vi "Write Cell Status File.vi"(7 "Cell Select":i32, 9 "GenInfoIn":T1, 10 "Test Info":T2 {"Cell Data"."Rw Temp" format="%.2f"; "Cell Data"."Rw" format="%.2f"; "Cell Data"."DAQ Units" items=["Mins", "Hrs"]; "Cell Data"."CurData" format="%.3f"; "Cell Data"."Last Pore Vol" format="%.3f"; "Cell Data"."Amplitude" format="%.3f"; "Cell Data"."ElectSpace" format="%.2f"; "Cell Data"."Permeability" format="%.2f"; "Cell Data"."Porosity" format="%.2f"; "Cell Data"."Diameter" format="%.2f"; "Cell Data"."Length" format="%.2f"}, 11 "Filepath":path) -> (3 "FilePathOut":path)   [LabVIEW 2013]
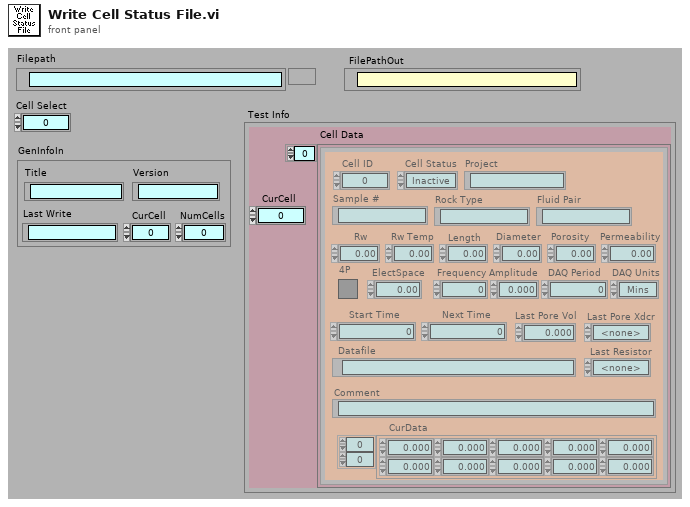
[diagram p1: front panel]
types:
  T1 = cluster{"Title":string, "Version":string, "Last Write":string, "CurCell":i32, "NumCells":i32}
  T2 = cluster{"CurCell":i32, "Cell Data":cluster{"Cell ID":i32, "Cell Status":enum16{"Inactive", "Setup", "Active", "Done"}, "Project":string, "Sample #":string, "Rock Type":string, "Fluid Pair":string, "Rw":dbl, "Rw Temp":dbl, "Length":dbl, "Diameter":dbl, "Porosity":dbl, "Permeability":dbl, "4P":bool, "ElectSpace":dbl, "Frequency":dbl, "Amplitude":dbl, "DAQ Period":u32, "DAQ Units":u16, "Start Time":dbl, "Next Time":dbl, "Datafile":path, "Last Pore Vol":dbl, "Last Pore Xdcr":enum16{"<none>", "Lo Range", "Hi Range"}, "Last Resistor":enum16{"<none>", "Resistor 1", "Resistor 2", "Resistor 3", "Resistor 4", "Resistor 5", "Resistor 6"}, "CurData":dbl[][], "Comment":string}[]}
  T3 = enum16{"New File", "Read Cell Status", "Write Cell Status"}
  T4 = cluster{"Cell ID":i32, "Cell Status":enum16{"Inactive", "Setup", "Active", "Done"}, "Project":string, "Sample #":string, "Rock Type":string, "Fluid Pair":string, "Rw":dbl, "Rw Temp":dbl, "Length":dbl, "Diameter":dbl, "Porosity":dbl, "Permeability":dbl, "4P":bool, "ElectSpace":dbl, "Frequency":dbl, "Amplitude":dbl, "DAQ Period":u32, "DAQ Units":u16, "Start Time":dbl, "Next Time":dbl, "Datafile":path, "Last Pore Vol":dbl, "Last Pore Xdcr":enum16{"<none>", "Lo Range", "Hi Range"}, "Last Resistor":enum16{"<none>", "Resistor 1", "Resistor 2", "Resistor 3", "Resistor 4", "Resistor 5", "Resistor 6"}, "CurData":dbl[][], "Comment":string}[]
  T5 = cluster{"Cell ID":i32, "Cell Status":enum16{"Inactive", "Setup", "Active", "Done"}, "Project":string, "Sample #":string, "Rock Type":string, "Fluid Pair":string, "Rw":dbl, "Rw Temp":dbl, "Length":dbl, "Diameter":dbl, "Porosity":dbl, "Permeability":dbl, "4P":bool, "ElectSpace":dbl, "Frequency":dbl, "Amplitude":dbl, "DAQ Period":u32, "DAQ Units":u16, "Start Time":dbl, "Next Time":dbl, "Datafile":path, "Last Pore Vol":dbl, "Last Pore Xdcr":enum16{"<none>", "Lo Range", "Hi Range"}, "Last Resistor":enum16{"<none>", "Resistor 1", "Resistor 2", "Resistor 3", "Resistor 4", "Resistor 5", "Resistor 6"}, "CurData":dbl[][], "Comment":string}
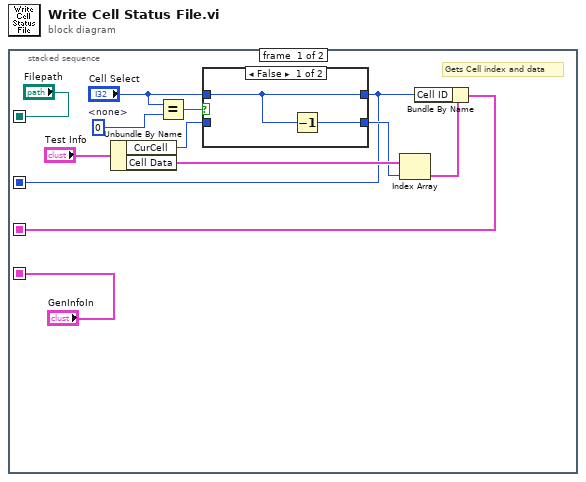
[diagram p0: block diagram]
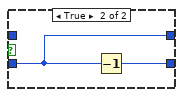
[diagram p2: hidden frame]
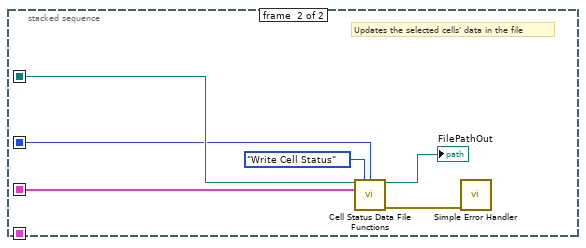
[diagram p3: hidden frame]
diagram:
  n1 = stacked-sequence {
    seq-local: ["Filepath" _] -> [_ w20]
    seq-local: [w7 _] -> [_ w21]
    seq-local: ["GenInfoIn" _] -> [_ _]
    seq-local: [w1 _] -> [_ w19]
    frame #0 {
      w2 = 0  # <none>
      # "Gets Cell index and data"
      n2 = Unbundle By Name("Test Info") -> ("CurCell"=w3:i32, "Cell Data"=w10:T4)
      n3 = Equal?(x="Cell Select", y=w2) -> (x = y?=w6:bool)
      n4 = case shown="False" w6 {
        tunnel: "Cell Select" -> [w14 _]
        tunnel: [w13 w15] -> w4
        tunnel: [w14 w16] -> w1
        tunnel: w3 -> [_ w16]
        frame False {
          n5 = Decrement(x=w14) -> (x-1=w13:i32)
        }
        frame True {
          n6 = Decrement(x=w16) -> (x-1=w15:i32)
        }
      }
      n7 = Index Array(array=w10, index=w4) -> (element=w8:T5)
      n8 = Bundle By Name(cluster=w8, "Cell ID"=w1) -> (w7:T5)
    }
    frame #1 {
      # "Updates the selected cells' data in the file"
      n9 = call "Cell Status Data File Functions.vi"("FilePathIn"=w20, "Function"=T3."Write Cell Status", "Cell Select - RO"=w19, "Cell x Data In"=w21) -> ("FilePathOut"=→"FilePathOut":path, "ErrorOut"=w18:errorcluster)  [unwired: 7 in, 3 out]
      n10 = call <vilib>:"Simple Error Handler.vi"("error in (no error)"=w18) -> ()  [unwired: 4 in, 5 out]
    }
  }
